vi "WritePosition.vi"(9 "Z":dbl, 10 "Y":dbl, 11 "X":dbl) -> ()   [LabVIEW 2017]
uses:
  Settings/Traverse-Settings-Global.vi
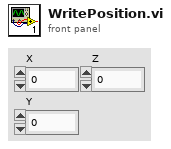
[diagram p1: front panel]
types:
  T1 = typedef "Settings-Control.ctl" = cluster{"Acceleration":dbl[], "Deceleration":dbl[], "Max Velocity":dbl[], "Speed":dbl, "Pulse/Degree":dbl, "Degre Factor":dbl[], "mm/rotation":dbl[], "Position":dbl[]}
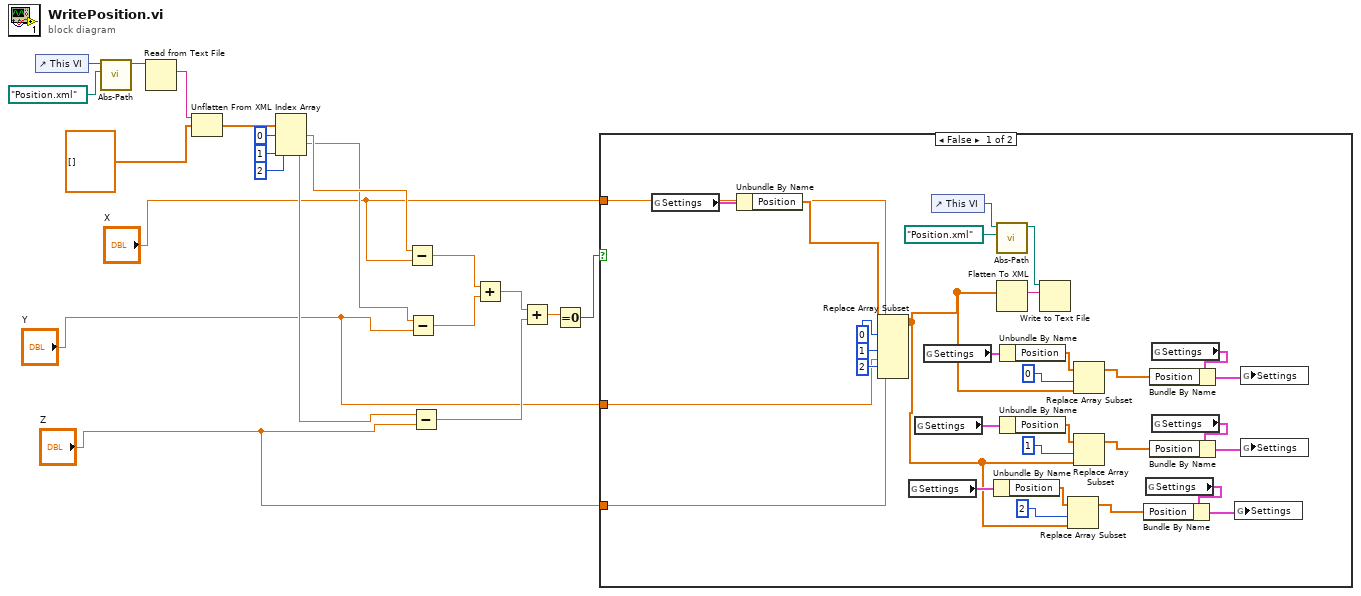
[diagram p0: block diagram]
diagram:
  n1 = control-ref of="This VI"() -> (w19:refnum<vi>)
  n2 = call "Abs-Path.vi"("filename"=path "Position.xml" ("file (use dialog)"), "Vi in path"=w19) -> ("Full path"=w18:path)  [unwired: 9 in]
  n3 = Read from Text File(file (use dialog)=w18) -> (text=w21:string)  [unwired: 3 in, 3 out]
  n4 = Unflatten From XML(xml string=w21, type=dbl[] [] ("Acceleration")) -> (value=w16:dbl[])  [unwired: 1 in, 1 out]
  n5 = Index Array(array=w16, index #1=0 ("index"), index #2=1 ("index"), index #3=2 ("index")) -> (element #1=w12:dbl, element #2=w11:dbl, element #3=w10:dbl)
  n6 = Subtract(x=w12, y="X") -> (x-y=w8:dbl)
  n7 = Subtract(x=w11, y="Y") -> (x-y=w9:dbl)
  n8 = Subtract(x=w10, y="Z") -> (x-y=w6:dbl)
  n9 = Add(x=w8, y=w9) -> (x+y=w7:dbl)
  n10 = Add(x=w7, y=w6) -> (x+y=w5:dbl)
  n11 = Equal To 0?(x=w5) -> (x = 0?=w4:bool)
  n12 = case shown="False" w4 {
    tunnel: "X" -> [w43 _]
    tunnel: "Y" -> [w42 _]
    tunnel: "Z" -> [w41 _]
    frame False {
      n13 = global read "Traverse-Settings-Global.vi" "Settings"() -> (w51:T1)
      n14 = Unbundle By Name(w51) -> ("Position"=w52:dbl[])
      n15 = Replace Array Subset(array=w52, new element #1=w43, index #1=0 ("index"), new element #2=w42, index #2=1 ("index"), new element #3=w41, index #3=2 ("index")) -> (w22:dbl[])
      n16 = global read "Traverse-Settings-Global.vi" "Settings"() -> (w26:T1)
      n17 = global read "Traverse-Settings-Global.vi" "Settings"() -> (w32:T1)
      n18 = global read "Traverse-Settings-Global.vi" "Settings"() -> (w38:T1)
      n19 = control-ref of="This VI"() -> (w49:refnum<vi>)
      n20 = Unbundle By Name(w26) -> ("Position"=w27:dbl[])
      n21 = call "Abs-Path.vi"("filename"=path "Position.xml" ("file (use dialog)"), "Vi in path"=w49) -> ("Full path"=w50:path)  [unwired: 9 in]
      n22 = Flatten To XML(anything=w22) -> (xml string=w48:string)
      n23 = Unbundle By Name(w38) -> ("Position"=w39:dbl[])
      n24 = Unbundle By Name(w32) -> ("Position"=w33:dbl[])
      n25 = Write to Text File(file (use dialog)=w50, text=w48) -> ()  [unwired: 2 in, 3 out]
      n26 = Replace Array Subset(array=w27, new element=w22, index=2) -> (w28:dbl[])
      n27 = Replace Array Subset(array=w39, new element=w22, index=0) -> (w40:dbl[])
      n28 = Replace Array Subset(array=w33, new element=w22, index=1) -> (w34:dbl[])
      n29 = global read "Traverse-Settings-Global.vi" "Settings"() -> (w25:T1)
      n30 = Bundle By Name(cluster=w25, "Position"=w28) -> (w24:T1)
      n31 = global read "Traverse-Settings-Global.vi" "Settings"() -> (w37:T1)
      n32 = Bundle By Name(cluster=w37, "Position"=w40) -> (w36:T1)
      n33 = global read "Traverse-Settings-Global.vi" "Settings"() -> (w31:T1)
      n34 = Bundle By Name(cluster=w31, "Position"=w34) -> (w30:T1)
      n35 = global write "Traverse-Settings-Global.vi" "Settings"(w24) -> ()
      n36 = global write "Traverse-Settings-Global.vi" "Settings"(w36) -> ()
      n37 = global write "Traverse-Settings-Global.vi" "Settings"(w30) -> ()
    }
    frame True {
    }
  }
